vi "LVClass_CameraSet Load UserParametersValue.vi"(0 "CameraSet.lvclass":refnum<class "CameraSet.lvclass">, 5 "ParametersValue file path":path, 11 "error in (no error)":errorcluster) -> (4 "CameraSet.lvclass":refnum<class "CameraSet.lvclass">, 15 "error out":errorcluster)   [LabVIEW 2020, in "CameraSet.lvclass"]
doc: "Load file content to CameraSet object.\n\n<B>CameraSetIn</B> : CameraSet object.\n<B>CameraSetOut</B> : CameraSet object.\n<B>file_path</B> : Absolute path to the file."
uses:
  CameraSet.lvclass
  CameraSet.lvclass/CameraSet.ctl
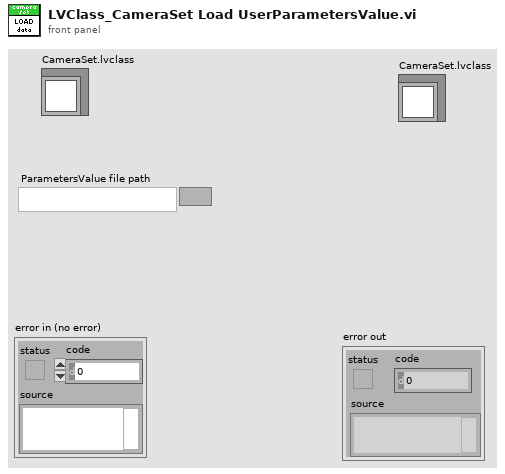
[diagram p1: front panel]
types:
  T1 = typedef "ClassID.ctl" = i64
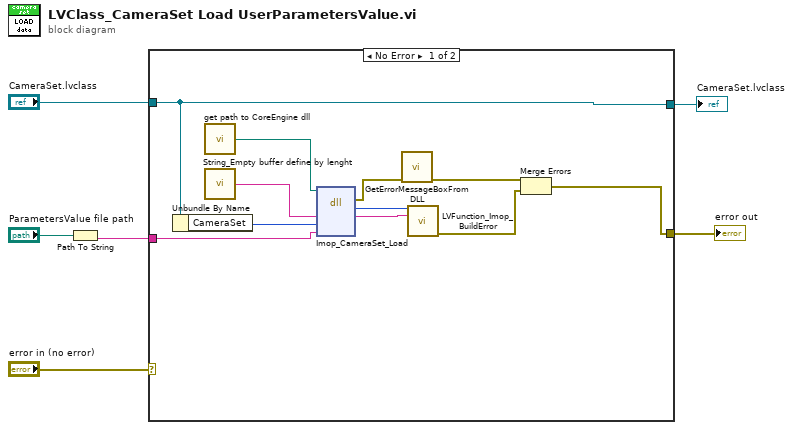
[diagram p0: block diagram]
diagram:
  n1 = Path To String(path="ParametersValue file path") -> (string=w4:string)
  n2 = case shown="No Error" "error in (no error)" {
    selector: "error in (no error)" -> [_ w18]
    tunnel: w4 -> [w14 _]
    tunnel: "CameraSet.lvclass" -> [w7 w19]
    tunnel: [w7 w19] -> w2
    tunnel: [w9 w18] -> w1
    frame No Error {
      n3 = Unbundle By Name(w7) -> ("CameraSet"=w8:T1)
      n4 = call "get path to CoreEngine dll.vi"() -> ("path to c_interface_vc100.dll"=w13:path)  [unwired: 12 in, 3 out]
      n5 = call "String_Empty buffer define by lenght.vi"() -> ("Empty buffer"=w17:string)  [unwired: 1 in]
      n6 = dll-call lib="D:/soft/HASO_v3/SVN_trunk/ImOpCoreEngine4_LV2011/DLLs/c_interface_vc100.dll" fn="Imop_CameraSet_Load"(path in=w13, "message"=w17, "objet"=w8, "chemin_config"=w14) -> (error out=w12:errorcluster, "return type"=w15:i32, "message"=w16:string)  [unwired: 4 in, 1 out]
      n7 = call "GetErrorMessageBoxFromDLL.vi"("error IN"=w12) -> ("error OUT"=w11:errorcluster)  [unwired: 10 in]
      n8 = call "LVFunction_Imop_BuildError.vi"("code"=w15, "String to Prepend to source (\"\")"=w16) -> ("error out"=w10:errorcluster)  [unwired: 13 in]
      n9 = Merge Errors(w11, w10) -> (w9:errorcluster)
    }
    frame Error {
    }
  }
  "CameraSet.lvclass" <- w2
  "error out" <- w1
